vi "Shooter Speed Control.vi"(8 "reinitialize? (F)":bool, 9 "full power":bool, 10 "Bottom RPM":dbl format="%.2f", 11 "Top RPM":dbl) -> ()   [LabVIEW 2011]
uses:
  <vilib>/addons/control/pid/pid.llb/PID (DBL).vi
  Robot Global Data.vi
  <vilib>/addons/control/pid/NI_PID_pid.lvlib
panel:
  in  "Bottom PID gains":T1={"proportional gain (Kc)"=6.0, "integral time (Ti, min)"=0.003, "derivative time (Td, min)"=0.0} {"derivative time (Td, min)" format="%.3f"; "integral time (Ti, min)" format="%.3f"; "proportional gain (Kc)" format="%.3f"}
  in  "Top PID gains":T1={"proportional gain (Kc)"=6.0, "integral time (Ti, min)"=0.003, "derivative time (Td, min)"=0.0} {"derivative time (Td, min)" format="%.3f"; "integral time (Ti, min)" format="%.3f"; "proportional gain (Kc)" format="%.3f"}
  out "Bottom RPM out":dbl(graph)
  out "Top RPM out":dbl(graph)
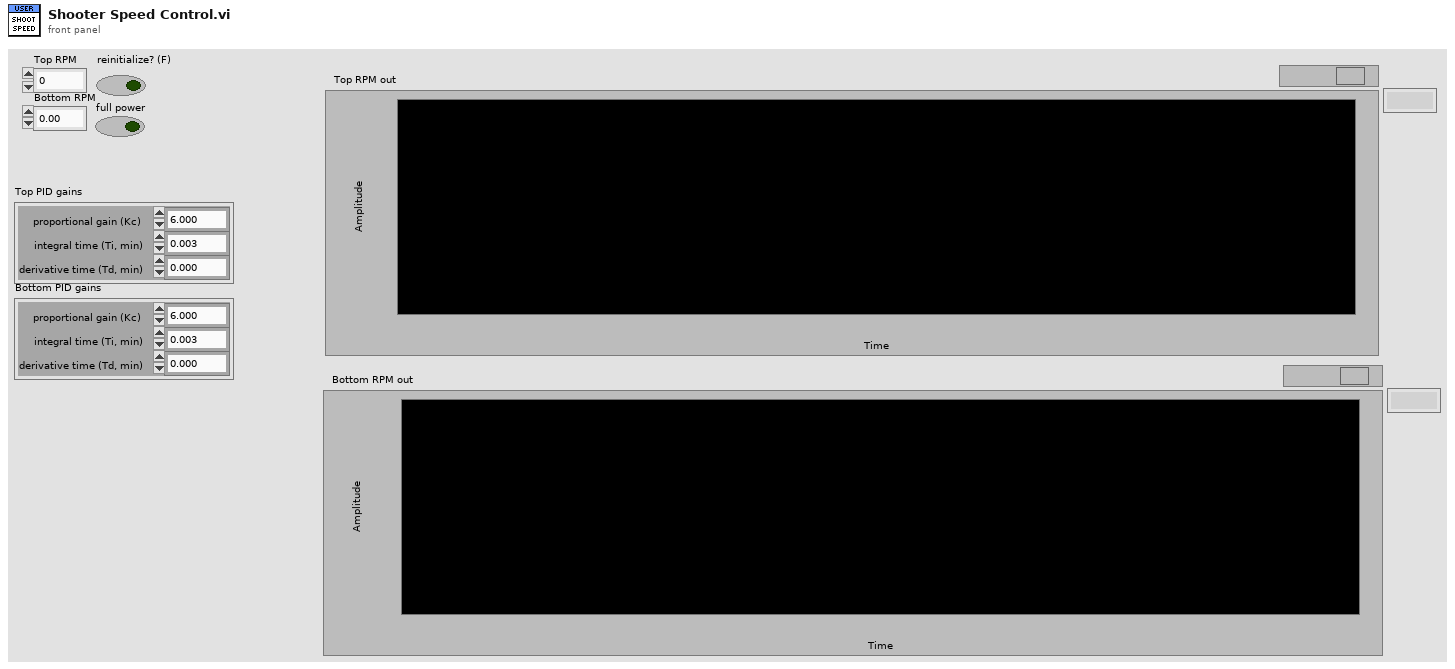
[diagram p1: front panel]
types:
  T1 = cluster{"proportional gain (Kc)":dbl, "integral time (Ti, min)":dbl, "derivative time (Td, min)":dbl}
  T2 = typedef "WPI_CounterDevRef.ctl" = cluster{"DevStatus":errorcluster, "CntIndex":T3}
  T3 = typedef "FPGA_CounterCtrSystemIndex.ctl" = enum8{"Ctr 0", "Ctr 1", "Ctr 2", "Ctr 3", "Ctr 4", "Ctr 5", "Ctr 6", "Ctr 7", "Invalid"}
  T4 = typedef "WPI_MotorControlDeviceRef.ctl" = cluster{"DeviceStatus":errorcluster, "Type":enum16{"PWM", "CAN"}, "PWM":cluster{"Digital Module":T5, "PWM Channel":T6, "DeadBand":T7}, "CAN":cluster{"Device Number":u8, "Control Mode":T8, "Semaphore":T9, "Max Vout":dbl}, "Invert":bool, "TransformRef":T10, "InvTransformRef":T10}
  T5 = typedef "FPGA_TypedefDigitalModule.ctl" = enum16{"Digital Module 1", "Digital Module 2"}
  T6 = typedef "FPGA_DIOPWMChannel.ctl" = enum8{"PWM 1", "PWM 2", "PWM 3", "PWM 4", "PWM 5", "PWM 6", "PWM 7", "PWM 8", "PWM 9", "PWM 10", "Invalid"}
  T7 = typedef "WPI_PWMDeadband.ctl" = cluster{"Name":string, "maxPositivePwm":i32, "minPositivePwm":i32, "centerPwm":i32, "maxNegativePwm":i32, "minNegativePwm":i32, "angularRange":u16}
  T8 = typedef "WPI_CANJaguar_ControlMode.ctl" = enum8{"Percent VBus", "Current", "Speed", "Position", "Voltage"}
  T9 = typedef "Semaphore RefNum" = refnum<k1>
  T10 = typedef "WPI_PWMTransform_ConPane.ctl" = refnum<vi>
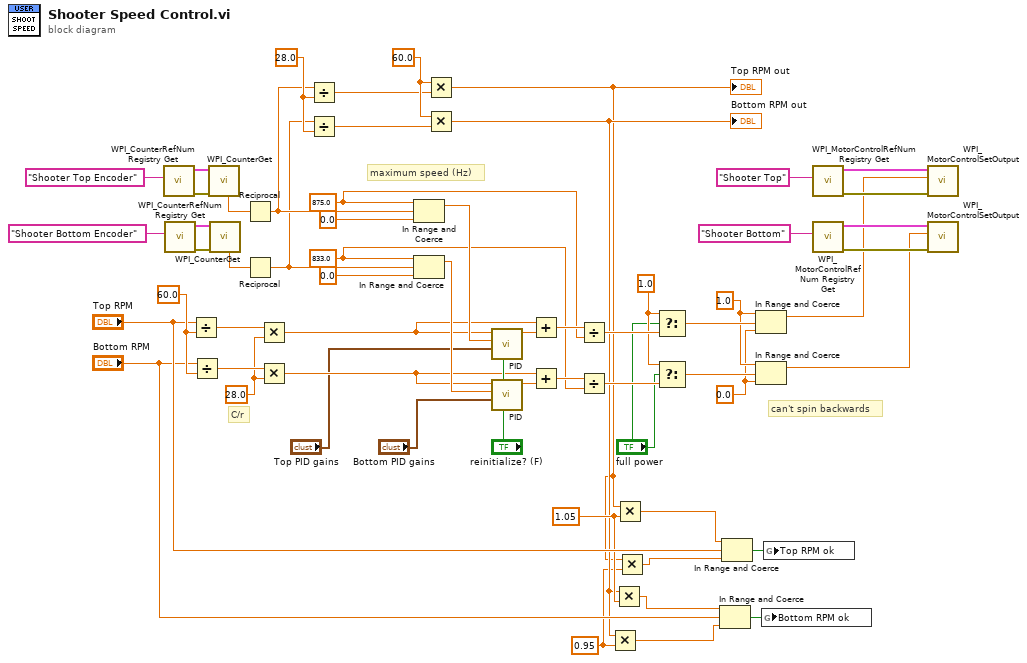
[diagram p0: block diagram]
diagram:
  w3 = 0.95 ("y")
  w7 = 1.05 ("y")
  w17 = 28.0 ("y")
  w20 = 60.0 ("x")
  w21 = 28.0 ("y")
  w26 = 60.0 ("y")
  w35 = 0.0 ("lower limit")
  w36 = 1.0 ("upper limit")
  w40 = 1.0 ("t")
  w30 = 833.0 ("upper limit")
  w43 = 875.0 ("upper limit")
  # "C/r"
  # "maximum speed (Hz)"
  # "can't spin backwards"
  n1 = call <vilib>:"WPI_CounterRefNum Registry Get.vi"("refnum name"="Shooter Top Encoder") -> ("error out"=w57:errorcluster, "CounterDevRef"=w56:T2)  [unwired: 9 in]
  n2 = call <vilib>:"WPI_CounterRefNum Registry Get.vi"("refnum name"="Shooter Bottom Encoder") -> ("error out"=w55:errorcluster, "CounterDevRef"=w54:T2)  [unwired: 9 in]
  n3 = Divide(x="Top RPM", y=w26) -> (x/y=w25:dbl)
  n4 = Divide(x="Bottom RPM", y=w26) -> (x/y=w24:dbl)
  n5 = call <vilib>:"WPI_CounterGet.vi"("error in (no error)"=w57, "CounterDevRef in"=w56) -> ("Period (sec)"=w53:dbl)  [unwired: 4 in, 5 out]
  n6 = call <vilib>:"WPI_CounterGet.vi"("error in (no error)"=w55, "CounterDevRef in"=w54) -> ("Period (sec)"=w52:dbl)  [unwired: 4 in, 5 out]
  n7 = Reciprocal(x=w53) -> (1/x=w16:dbl)
  n8 = Reciprocal(x=w52) -> (1/x=w15:dbl)
  n9 = Multiply(x=w25, y=w21) -> (x*y=w22:dbl)
  n10 = Multiply(x=w24, y=w21) -> (x*y=w23:dbl)
  n11 = Divide(x=w16, y=w17) -> (x/y=w19:dbl)
  n12 = Divide(x=w15, y=w17) -> (x/y=w18:dbl)
  n13 = In Range and Coerce(upper limit=w43, x=w16, lower limit=0.0) -> (coerced(x)=w33:dbl)  [unwired: 1 out]
  n14 = In Range and Coerce(upper limit=w30, x=w15, lower limit=0.0) -> (coerced(x)=w34:dbl)  [unwired: 1 out]
  n15 = Multiply(x=w20, y=w19) -> (x*y=w2:dbl)
  "Top RPM out" <- w2
  n16 = Multiply(x=w20, y=w18) -> (x*y=w4:dbl)
  "Bottom RPM out" <- w4
  n17 = call-poly <vilib>:"PID.vi"("reinitialize? (F)"="reinitialize? (F)", "PID gains"="Top PID gains", "process variable"=w33, "setpoint"=w22) -> ("output"=w32:dbl)  [unwired: 6 in, 1 out]
  n18 = call-poly <vilib>:"PID.vi"("reinitialize? (F)"="reinitialize? (F)", "PID gains"="Bottom PID gains", "process variable"=w34, "setpoint"=w23) -> ("output"=w31:dbl)  [unwired: 6 in, 1 out]
  n19 = Add(x=w22, y=w32) -> (x+y=w47:dbl)
  n20 = Add(x=w23, y=w31) -> (x+y=w46:dbl)
  n21 = Divide(x=w47, y=w43) -> (x/y=w41:dbl)
  n22 = Divide(x=w46, y=w30) -> (x/y=w42:dbl)
  n23 = Multiply(x=w4, y=w3) -> (x*y=w5:dbl)
  n24 = Multiply(x=w4, y=w7) -> (x*y=w6:dbl)
  n25 = Multiply(x=w2, y=w7) -> (x*y=w8:dbl)
  n26 = Multiply(x=w2, y=w3) -> (x*y=w1:dbl)
  n27 = Select(t=w40, s="full power", f=w41) -> (s? t:f=w39:dbl)
  n28 = Select(t=w40, s="full power", f=w42) -> (s? t:f=w37:dbl)
  n29 = In Range and Coerce(upper limit=w6, x="Bottom RPM", lower limit=w5) -> (In Range?=w12:bool)  [unwired: 1 out]
  n30 = In Range and Coerce(upper limit=w8, x="Top RPM", lower limit=w1) -> (In Range?=w11:bool)  [unwired: 1 out]
  n31 = In Range and Coerce(upper limit=w36, x=w39, lower limit=w35) -> (coerced(x)=w38:dbl)  [unwired: 1 out]
  n32 = In Range and Coerce(upper limit=w36, x=w37, lower limit=w35) -> (coerced(x)=w27:dbl)  [unwired: 1 out]
  n33 = global write "Robot Global Data.vi" "Bottom RPM ok"(w12) -> ()
  n34 = global write "Robot Global Data.vi" "Top RPM ok"(w11) -> ()
  n35 = call <vilib>:"WPI_MotorControlRefNum Registry Get.vi"("refnum name"="Shooter Top") -> ("error out"=w50:errorcluster, "MotorControlDevRef"=w51:T4)  [unwired: 9 in]
  n36 = call <vilib>:"WPI_MotorControlRefNum Registry Get.vi"("refnum name"="Shooter Bottom") -> ("error out"=w48:errorcluster, "MotorControlDevRef"=w49:T4)  [unwired: 9 in]
  n37 = call <vilib>:"WPI_MotorControlSetOutput.vi"("error in (no error)"=w50, "Output"=w38, "MotorControlDevRef"=w51) -> ()  [unwired: 7 in, 2 out]
  n38 = call <vilib>:"WPI_MotorControlSetOutput.vi"("error in (no error)"=w48, "Output"=w27, "MotorControlDevRef"=w49) -> ()  [unwired: 7 in, 2 out]
